vi "Enqueue Error.vi"(8 "Error-Enqueuer in":T1, 11 "error in (no error)":errorcluster) -> (0 "Error-Enqueuer out":T1, 3 "error out":errorcluster)   [LabVIEW 2018, in "Scripting.lvlib" / "Actor.lvclass"]
uses:
  Actor.lvclass
  Internal-Enqueuers.ctl
  Internal-Stop.ctl
  Internal-Error.ctl
  <vilib>/event_ctls.llb/usereventprio.ctl
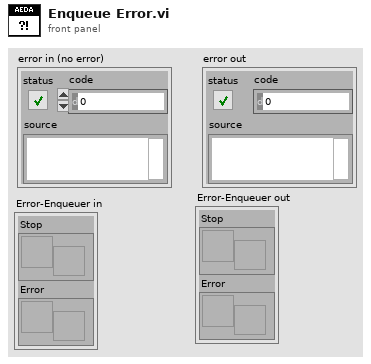
[diagram p1: front panel]
types:
  T1 = typedef "Scripting.lvlib/Actor.lvclass/Internal-Enqueuers.ctl" = cluster{"Stop":refnum<user-event>, "Error":refnum<user-event>}
  T2 = typedef "Scripting.lvlib/Actor.lvclass/Internal-Error.ctl" = cluster{"Error":errorcluster}
  T3 = typedef "usereventprio.ctl" = enum32{"high priority", "normal priority"}
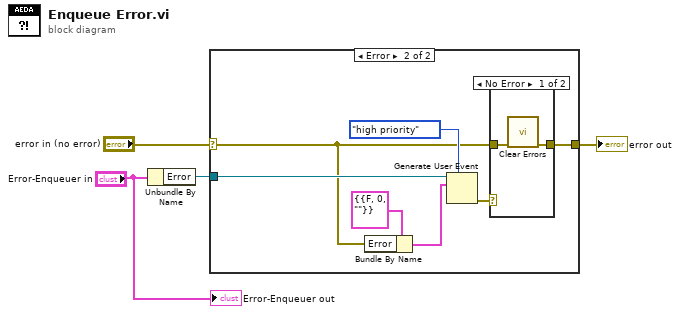
[diagram p0: block diagram]
diagram:
  n1 = Unbundle By Name("Error-Enqueuer in") -> ("Error"=w1:refnum<user-event>)
  n2 = case shown="Error" "error in (no error)" {
    selector: "error in (no error)" -> [w5 w6]
    tunnel: [w5 w11] -> w4
    tunnel: w1 -> [_ w9]
    frame No Error {
    }
    frame Error {
      n3 = Bundle By Name(cluster=T2 {"Error"={"status"=FALSE, "code"=0, "source"=""}} ("event data"), "Error"=w6) -> (w7:T2)
      n4 = Generate User Event(priority (normal)=usereventprio."high priority", user event=w9, event data cluster=w7) -> (error out=w12:errorcluster)  [unwired: 1 in, 1 out]
      n5 = case shown="No Error" w12 {
        tunnel: [w14 w15] -> w11
        tunnel: w6 -> [w13 w15]
        frame No Error {
          n6 = call <vilib>:"Clear Errors.vi"("error in (no error)"=w13) -> ("error out"=w14:errorcluster)  [unwired: 5 in, 1 out]
        }
        frame Error {
        }
      }
    }
  }
  "error out" <- w4
  "Error-Enqueuer out" <- "Error-Enqueuer in"
